vi "PasteFits.vi"(6 "Clipboard":refnum<vi>, 8 "error in (no error)":errorcluster, 10 "Cell Start":T1, 11 "Table CtlRef In":refnum<vi>) -> (0 "error out":errorcluster, 1 "Clipboard (clipped)":string[][](array[string]), 2 "Paste Fits?":bool, 3 "Table CtlRef Out":refnum<vi>)   [LabVIEW 2013]
uses:
  <vilib>/Utility/miscctls.llb/LVRowAndColumnTypeDef.ctl
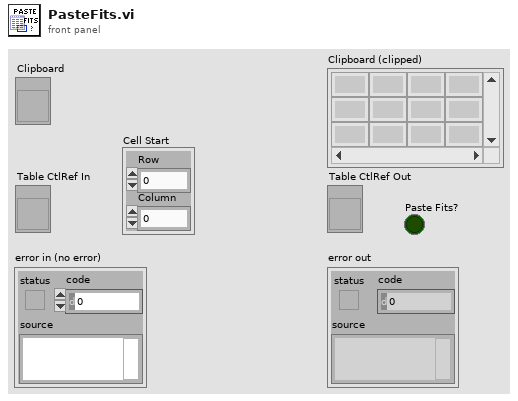
[diagram p1: front panel]
types:
  T1 = typedef "LVRowAndColumnTypeDef.ctl" = cluster{"Row":i32, "Column":i32}
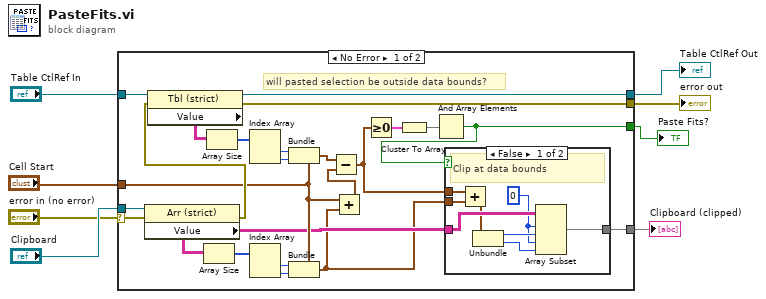
[diagram p0: block diagram]
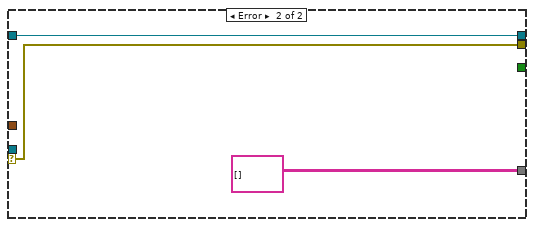
[diagram p3: hidden frame]
diagram:
  n1 = case shown="No Error" "error in (no error)" {
    selector: "error in (no error)" -> [w17 w42]
    tunnel: "Cell Start" -> [w22 _]
    tunnel: "Table CtlRef In" -> [w21 w43]
    tunnel: "Clipboard" -> [w20 _]
    tunnel: [w19 w43] -> w5
    tunnel: [w18 w42] -> w4
    tunnel: [w12 _] -> w3
    tunnel: [w13 string[][] [] ("Clipboard 2")] -> w1
    frame No Error {
      # "will pasted selection be outside data bounds?"
      n2 = property class="Arr (strict)"(reference=w20, error in=w17) -> (error out=w26:errorcluster, "Value"=w14:string[][])  [unwired: 1 out]
      n3 = property class="Tbl (strict)"(reference=w21, error in=w26) -> (reference out=w19:refnum<vi>, error out=w18:errorcluster, "Value"=w23:string[][])
      n4 = Array Size(array=w14) -> (size(s)=w31:i32[])
      n5 = Array Size(array=w23) -> (size(s)=w29:i32[])
      n6 = Index Array(array=w29) -> (element #1=w28:i32, element #2=w27:i32)  [unwired: 2 in]
      n7 = Index Array(array=w31) -> (element #1=w30:i32, element #2=w9:i32)  [unwired: 2 in]
      n8 = Bundle(cluster=w22, "Row"=w28, "Column"=w27) -> (w25:T1)
      n9 = Bundle(cluster=w22, "Row"=w30, "Column"=w9) -> (w10:T1)
      n10 = Add(x=w22, y=w10) -> (x+y=w24:T1)
      n11 = Subtract(x=w25, y=w24) -> (x-y=w11:T1)
      n12 = Greater Or Equal To 0?(x=w11) -> (x >= 0?=w16:cluster{"Row":bool, "Column":bool})
      n13 = Cluster To Array(cluster=w16) -> (array=w15:bool[])
      n14 = And Array Elements(Boolean array=w15) -> (logical AND=w12:bool)
      n15 = case shown="False" w12 {
        tunnel: w14 -> [w37 w40]
        tunnel: [w36 w40] -> w13
        tunnel: w11 -> [w39 _]
        tunnel: w10 -> [w38 _]
        frame False {
          w32 = 0 ("index")
          # "Clip at data bounds"
          n16 = Add(x=w39, y=w38) -> (x+y=w35:T1)
          n17 = Unbundle(w35) -> ("Row"=w33:i32, "Column"=w34:i32)
          n18 = Array Subset(array=w37, index (row)=w32, length (row)=w33, index (col)=w32, length (col)=w34) -> (w36:string[][])
        }
        frame True {
          # "Paste Area OK!"
        }
      }
    }
    frame Error {
    }
  }
  "error out" <- w4
  "Table CtlRef Out" <- w5
  "Paste Fits?" <- w3
  "Clipboard (clipped)" <- w1
